vi "LSMcontroller_v57.vi"() -> ()   [LabVIEW 2015] (continued)
                    n4617 = local read "maxbufferAI"() -> (w1341:i32)
                    n4618 = local read "Override AI buffer"() -> (w1337:bool)
                    n4619 = call "2pparameters.vi"("command"="get") -> ("params out"=w1354:T12)  [unwired: 1 in]
                    n4620 = Bundle By Name(cluster=w1354, "type"="X-Y-t movie", "avpp"=w1357, "Angle Img"=w1356, "Xpixels Img"=w1352, "Vx-min Img"=w1351, "VX-max Img"=w1350, "Ypixels Img"=w1348, "Vy-min Img"=w1349, "Vy-max Img"=w1345, "srate"=w1339, "srate Img"=w1339, "finite"=w1340, "cont"=w1343, "wavdet"=w1344, "measpoints"=w1342, "maxbufferAI"=w1341, "Drawing Mode"=w1355, "Vz-reset"=0.0, "AIoverride"=w1337) -> (w1346:T12)
                    n4621 = call "2pparameters.vi"("Params in"=w1346, "command"="set") -> ()  [unwired: 1 out]
                  }
                  frame "X-Y-Z stack" {
                    n4622 = call "2pparameters.vi"("command"="get") -> ("params out"=w1361:T12)  [unwired: 1 in]
                    n4623 = Bundle By Name(cluster=w1361, "type"="X-Y-Z stack") -> (w1359:T12)
                    n4624 = call "2pparameters.vi"("Params in"=w1359, "command"="set") -> ()  [unwired: 1 out]
                  }
                  frame "Lifetime (scan)" {
                    n4625 = call "2pparameters.vi"("command"="get") -> ("params out"=w1366:T12)  [unwired: 1 in]
                    n4626 = Bundle By Name(cluster=w1366, "type"="Lifetime (scan)") -> (w1364:T12)
                    n4627 = call "2pparameters.vi"("Params in"=w1364, "command"="set") -> ()  [unwired: 1 out]
                  }
                  frame "Lifetime (contour)" {
                    n4628 = local read "Vy-min draw"() -> (w1376:dbl)
                    n4629 = local read "Vy-max draw"() -> (w1375:dbl)
                    n4630 = local read "Vx-min draw"() -> (w1378:dbl)
                    n4631 = local read "Vx-max draw"() -> (w1377:dbl)
                    n4632 = local read "xpixels ref"() -> (w1374:i32)
                    n4633 = local read "ypixels ref"() -> (w1373:i32)
                    n4634 = local read "ROI Type"() -> (w1372:u16)
                    n4635 = local read "srateAODOtt"() -> (w1383:dbl)
                    n4636 = local read "# of frames"() -> (w1388:i32)
                    n4637 = local read "refreshtime"() -> (w1380:dbl)
                    n4638 = local read "Pel"() -> (w1371:dbl)
                    n4639 = local read "bin"() -> (w1386:dbl)
                    n4640 = local read "Override AI buffer"() -> (w1369:bool)
                    n4641 = local read "finite samples"() -> (w1395:bool)
                    n4642 = local read "srateAODOtt"() -> (w1382:dbl)
                    n4643 = local read "srateAODOtt"() -> (w1389:dbl)
                    n4644 = local read "continuous"() -> (w1394:bool)
                    n4645 = local read "Angle ref"() -> (w1379:dbl)
                    n4646 = local read "wavdet"() -> (w1396:bool)
                    n4647 = local read "Vx-ref"() -> (w1391:dbl)
                    n4648 = local read "Vy-ref"() -> (w1393:dbl)
                    n4649 = local read "avpp"() -> (w1392:i32)
                    n4650 = call "tt_timeandsamples.vi"("bin"=w1386, "refreshtime"=w1380, "srateAODOtt"=w1383, "tot#ofsamples"=w1388) -> ("refreshrate"=w1384:dbl, "refreshbuffer"=w1385:i32, "timetracecycles"=w1390:i32)  [unwired: 5 in]
                    n4651 = local read "bin"() -> (w1387:dbl)
                    n4652 = call "2pparameters.vi"("command"="get") -> ("params out"=w1399:T12)  [unwired: 1 in]
                    n4653 = Bundle By Name(cluster=w1399, "Drawing Mode"=w1372, "measpoints"=w1388, "tt_cycles"=w1390, "refreshbuffer"=w1385, "refreshrate"=w1384, "Vx-ref"=w1391, "Vy-ref"=w1393, "srate"=w1382, "finite"=w1395, "cont"=w1394, "wavdet"=w1396, "avpp"=w1392, "srateAODO"=w1389, "bufferAI"=w1385, "bin"=w1387, "Angle Img"=w1379, "Vxminref"=w1378, "Vxmaxref"=w1377, "Vyminref"=w1376, "Vymaxref"=w1375, "Xpixels Img"=w1374, "Ypixels Img"=w1373, "Pel"=w1371, "Vz-reset"=0.0, "AIoverride"=w1369, "type"="Lifetime (contour)") -> (w1397:T12)
                    n4654 = Reciprocal(x=w1384) -> (1/x=w1381:dbl)
                    n4655 = local write "refreshtime"(w1381) -> ()
                    n4656 = call "2pparameters.vi"("Params in"=w1397, "command"="set") -> ()  [unwired: 1 out]
                  }
                  frame "X-Y-Z-t movie" {
                  }
                  frame "linescan" {
                  }
                  frame "Timetrace" {
                    n4657 = local read "Vy-min draw"() -> (w1409:dbl)
                    n4658 = local read "Vy-max draw"() -> (w1408:dbl)
                    n4659 = local read "Vx-min draw"() -> (w1411:dbl)
                    n4660 = local read "Vx-max draw"() -> (w1410:dbl)
                    n4661 = local read "xpixels ref"() -> (w1407:i32)
                    n4662 = local read "ypixels ref"() -> (w1406:i32)
                    n4663 = local read "ROI Type"() -> (w1405:u16)
                    n4664 = local read "srateAODOtt"() -> (w1416:dbl)
                    n4665 = local read "# of frames"() -> (w1421:i32)
                    n4666 = local read "refreshtime"() -> (w1413:dbl)
                    n4667 = local read "Pel"() -> (w1404:dbl)
                    n4668 = local read "bin"() -> (w1419:dbl)
                    n4669 = local read "Override AI buffer"() -> (w1402:bool)
                    n4670 = local read "finite samples"() -> (w1428:bool)
                    n4671 = local read "srateAODOtt"() -> (w1415:dbl)
                    n4672 = local read "srateAODOtt"() -> (w1422:dbl)
                    n4673 = local read "continuous"() -> (w1427:bool)
                    n4674 = local read "Angle ref"() -> (w1412:dbl)
                    n4675 = local read "wavdet"() -> (w1429:bool)
                    n4676 = local read "Vx-ref"() -> (w1424:dbl)
                    n4677 = local read "Vy-ref"() -> (w1426:dbl)
                    n4678 = local read "avpp"() -> (w1425:i32)
                    n4679 = call "tt_timeandsamples.vi"("bin"=w1419, "refreshtime"=w1413, "srateAODOtt"=w1416, "tot#ofsamples"=w1421) -> ("refreshrate"=w1417:dbl, "refreshbuffer"=w1418:i32, "timetracecycles"=w1423:i32)  [unwired: 5 in]
                    n4680 = local read "bin"() -> (w1420:dbl)
                    n4681 = call "2pparameters.vi"("command"="get") -> ("params out"=w1432:T12)  [unwired: 1 in]
                    n4682 = Bundle By Name(cluster=w1432, "Drawing Mode"=w1405, "measpoints"=w1421, "tt_cycles"=w1423, "refreshbuffer"=w1418, "refreshrate"=w1417, "Vx-ref"=w1424, "Vy-ref"=w1426, "srate"=w1415, "finite"=w1428, "cont"=w1427, "wavdet"=w1429, "avpp"=w1425, "srateAODO"=w1422, "bufferAI"=w1418, "bin"=w1420, "Angle Img"=w1412, "Vxminref"=w1411, "Vxmaxref"=w1410, "Vyminref"=w1409, "Vymaxref"=w1408, "Xpixels Img"=w1407, "Ypixels Img"=w1406, "Pel"=w1404, "Vz-reset"=0.0, "AIoverride"=w1402, "type"="Timetrace") -> (w1430:T12)
                    n4683 = Reciprocal(x=w1417) -> (1/x=w1414:dbl)
                    n4684 = local write "refreshtime"(w1414) -> ()
                    n4685 = call "2pparameters.vi"("Params in"=w1430, "command"="set") -> ()  [unwired: 1 out]
                  }
                  frame "Lifetime (point)" {
                  }
                }
              }
              frame #1 {
                w1435 = FALSE ("wavdet")
                n4686 = call "2pparameters.vi"("command"="get") -> ("params out"=w1439:T12)  [unwired: 1 in]
                n4687 = Bundle By Name(cluster=w1439, "finite"=w1435, "cont"=w1435, "wavdet"=TRUE) -> (w1436:T12)
                n4688 = call "2pparameters.vi"("Params in"=w1436, "command"="set") -> ()  [unwired: 1 out]
              }
              frame #2 {
                n4689 = local read "AO channels"() -> (w1444:u32)
                n4690 = call "2pparameters.vi"("command"="get") -> ("params out"=w1446:T12)  [unwired: 1 in]
                n4691 = Unbundle By Name(w1446) -> ("aAO"=w1445:u32[])
                n4692 = Search 1D Array(1D array=w1445, element=w1444) -> (index of element=w1442:i32)  [unwired: 1 in]
                n4693 = Greater?(x=w1442, y=-1) -> (0:w1441:bool)
                n4694 = case shown="True" w1441 {
                  tunnel: w1442 -> [_ w1456]
                  frame False {
                  }
                  frame True {
                    n4695 = local read "Meastab"() -> (w1449:enum32{"X-Y Image", "Linescan", "Timetrace"})
                    n4696 = local read "Tri padding value"() -> (w1450:dbl)
                    n4697 = local read "Amplitude (V)"() -> (w1454:dbl)
                    n4698 = local read "Tri Phase (s)"() -> (w1451:dbl)
                    n4699 = local read "Tri Repeats"() -> (w1452:dbl)
                    n4700 = local read "Frequency"() -> (w1453:dbl)
                    n4701 = local read "Offset (V)"() -> (w1455:dbl)
                    n4702 = case shown="\"Timetrace\"" w1449 {
                      tunnel: [w1457 w1458] -> w1448
                      frame "X-Y Image", Default {
                        n4703 = local read "Sampling rate"() -> (w1457:dbl)
                      }
                      frame "Timetrace" {
                        n4704 = local read "srateAODOtt"() -> (w1458:dbl)
                      }
                    }
                    n4705 = call "replace AO tri wf param.vi"("padding value"=w1450, "index of AO wave"=w1456, "Tri phase"=w1451, "Sampling frequency (Hz)"=w1448, "Tri Repeats"=w1452, "Frequency"=w1453, "Amplitude (V)"=w1454, "Offset (V)"=w1455) -> ()
                  }
                }
              }
              frame #3 {
                n4706 = case shown="True" w1459 {
                  tunnel: w1460 -> [_ w1469]
                  frame False {
                  }
                  frame True {
                    n4707 = call "waveformparamsv2.vi"("command"="get") -> ("Params out"=w1482:T16)  [unwired: 4 in, 2 out]
                    n4708 = Unbundle By Name(w1482) -> ("AO parameters"=w1481:T17)
                    n4709 = local read "Meastab"() -> (w1464:enum32{"X-Y Image", "Linescan", "Timetrace"})
                    n4710 = case shown="\"Timetrace\"" w1464 {
                      tunnel: [w1484 w1485] -> w1463
                      frame "X-Y Image", Default {
                        n4711 = local read "Sampling rate"() -> (w1484:dbl)
                      }
                      frame "Timetrace" {
                        n4712 = local read "srateAODOtt"() -> (w1485:dbl)
                      }
                    }
                    n4713 = Index Array(array=w1481, index=w1469) -> (element=w1471:T18)
                    n4714 = call "waveformsAObuffer.vi"("command"="get") -> ("AO wf out"=w1470:waveform(dbl)[])  [unwired: 1 in]
                    n4715 = call "generateTriWave_fromAOparameters.vi"("AO params"=w1471) -> ("Waveform"=w1468:waveform(dbl))  [unwired: 1 out]
                    n4716 = property on="refwf" class="Ring (strict)"() -> ("RingText.Text"=w1472:string)  [unwired: 2 in, 2 out]
                    n4717 = Replace Array Subset(array=w1470, new element=w1468, index=w1469) -> (w1467:waveform(dbl)[])
                    n4718 = call "waveformsDObuffer.vi"("command"="get") -> ("DO wf out"=w1477:digitalwaveform[])  [unwired: 1 in]
                    n4719 = call "correctwaveformsizetemp.vi"("new sampling frequency (Hz)"=w1463, "start"=FALSE, "reference waveforms to"=w1472, "Analog waveforms in"=w1467, "stop"=FALSE, "Digital waveforms in"=w1477) -> ("analog wf out"=w1475:waveform(dbl)[], "Digital wf out"=w1473:digitalwaveform[], "measpoints"=w1465:i32)
                    n4720 = local read "wavdet"() -> (w1466:bool)
                    n4721 = local write "Analog Lines Plot"(w1475) -> ()
                    n4722 = call "GetNumCamFramesv2.vi"("Digital Waveform Graph"=w1473) -> ("Numeric"=w1474:i32)  [unwired: 10 in]
                    n4723 = local write "Digital Lines Plot"(w1473) -> ()
                    n4724 = call "waveformsAObuffer.vi"("AO wf in"=w1475, "command"="set") -> ()  [unwired: 1 out]
                    n4725 = call "waveformsDObuffer.vi"("DO wf in"=w1473, "command"="set") -> ()  [unwired: 1 out]
                    n4726 = local write "Total Camera Frames"(w1474) -> ()
                    n4727 = case shown="True" w1466 {
                      tunnel: w1465 -> [_ w1486]
                      frame False {
                      }
                      frame True {
                        n4728 = local write "# of frames"(w1486) -> ()
                      }
                    }
                  }
                }
              }
              frame #4 {
                n4729 = local read "finite samples"() -> (w1487:bool)
                n4730 = local read "continuous"() -> (w1488:bool)
                n4731 = local read "wavdet"() -> (w1489:bool)
                n4732 = call "2pparameters.vi"("command"="get") -> ("params out"=w1492:T12)  [unwired: 1 in]
                n4733 = Bundle By Name(cluster=w1492, "finite"=w1487, "cont"=w1488, "wavdet"=w1489) -> (w1490:T12)
                n4734 = call "2pparameters.vi"("Params in"=w1490, "command"="set") -> ()  [unwired: 1 out]
              }
            }
          }
          event "Load Matlab Waveform": Value Change {
            n4735 = event-data() -> ()  [unwired: 1 in, 6 out]
            n4736 = stacked-sequence {
              seq-local: [_ _ w1600 _ _] -> [_ _ _ w1615 _]
              seq-local: [_ _ w1599 _ _] -> [_ _ _ w1614 _]
              frame #0 {
                n4737 = local read "Measurement"() -> (w1494:T5)
                n4738 = case shown="\"X-Y-t movie\", Default" w1494 {
                  frame "X-Y-t movie", Default {
                    n4739 = local read "avpp"() -> (w1515:i32)
                    n4740 = local read "Angle ref"() -> (w1514:dbl)
                    n4741 = local read "ROI Type"() -> (w1513:u16)
                    n4742 = local read "xpixels ref"() -> (w1510:i32)
                    n4743 = local read "Vx-min ref"() -> (w1509:dbl)
                    n4744 = local read "Vx-max ref"() -> (w1508:dbl)
                    n4745 = local read "ypixels ref"() -> (w1506:i32)
                    n4746 = local read "Vy-min ref"() -> (w1507:dbl)
                    n4747 = local read "Vy-max ref"() -> (w1503:dbl)
                    n4748 = local read "Sampling rate"() -> (w1497:dbl)
                    n4749 = local read "finite samples"() -> (w1498:bool)
                    n4750 = local read "continuous"() -> (w1501:bool)
                    n4751 = local read "wavdet"() -> (w1502:bool)
                    n4752 = local read "# of frames"() -> (w1500:i32)
                    n4753 = local read "maxbufferAI"() -> (w1499:i32)
                    n4754 = local read "Override AI buffer"() -> (w1495:bool)
                    n4755 = call "2pparameters.vi"("command"="get") -> ("params out"=w1512:T12)  [unwired: 1 in]
                    n4756 = Bundle By Name(cluster=w1512, "type"="X-Y-t movie", "avpp"=w1515, "Angle Img"=w1514, "Xpixels Img"=w1510, "Vx-min Img"=w1509, "VX-max Img"=w1508, "Ypixels Img"=w1506, "Vy-min Img"=w1507, "Vy-max Img"=w1503, "srate"=w1497, "srate Img"=w1497, "finite"=w1498, "cont"=w1501, "wavdet"=w1502, "measpoints"=w1500, "maxbufferAI"=w1499, "Drawing Mode"=w1513, "Vz-reset"=0.0, "AIoverride"=w1495) -> (w1504:T12)
                    n4757 = call "2pparameters.vi"("Params in"=w1504, "command"="set") -> ()  [unwired: 1 out]
                  }
                  frame "X-Y-Z stack" {
                    n4758 = call "2pparameters.vi"("command"="get") -> ("params out"=w1519:T12)  [unwired: 1 in]
                    n4759 = Bundle By Name(cluster=w1519, "type"="X-Y-Z stack") -> (w1517:T12)
                    n4760 = call "2pparameters.vi"("Params in"=w1517, "command"="set") -> ()  [unwired: 1 out]
                  }
                  frame "Lifetime (scan)" {
                    n4761 = call "2pparameters.vi"("command"="get") -> ("params out"=w1524:T12)  [unwired: 1 in]
                    n4762 = Bundle By Name(cluster=w1524, "type"="Lifetime (scan)") -> (w1522:T12)
                    n4763 = call "2pparameters.vi"("Params in"=w1522, "command"="set") -> ()  [unwired: 1 out]
                  }
                  frame "Lifetime (contour)" {
                    n4764 = local read "Vy-min draw"() -> (w1534:dbl)
                    n4765 = local read "Vy-max draw"() -> (w1533:dbl)
                    n4766 = local read "Vx-min draw"() -> (w1536:dbl)
                    n4767 = local read "Vx-max draw"() -> (w1535:dbl)
                    n4768 = local read "xpixels ref"() -> (w1532:i32)
                    n4769 = local read "ypixels ref"() -> (w1531:i32)
                    n4770 = local read "ROI Type"() -> (w1530:u16)
                    n4771 = local read "srateAODOtt"() -> (w1541:dbl)
                    n4772 = local read "# of frames"() -> (w1546:i32)
                    n4773 = local read "refreshtime"() -> (w1538:dbl)
                    n4774 = local read "Pel"() -> (w1529:dbl)
                    n4775 = local read "bin"() -> (w1544:dbl)
                    n4776 = local read "Override AI buffer"() -> (w1527:bool)
                    n4777 = local read "finite samples"() -> (w1553:bool)
                    n4778 = local read "srateAODOtt"() -> (w1540:dbl)
                    n4779 = local read "srateAODOtt"() -> (w1547:dbl)
                    n4780 = local read "continuous"() -> (w1552:bool)
                    n4781 = local read "Angle ref"() -> (w1537:dbl)
                    n4782 = local read "wavdet"() -> (w1554:bool)
                    n4783 = local read "Vx-ref"() -> (w1549:dbl)
                    n4784 = local read "Vy-ref"() -> (w1551:dbl)
                    n4785 = local read "avpp"() -> (w1550:i32)
                    n4786 = call "tt_timeandsamples.vi"("bin"=w1544, "refreshtime"=w1538, "srateAODOtt"=w1541, "tot#ofsamples"=w1546) -> ("refreshrate"=w1542:dbl, "refreshbuffer"=w1543:i32, "timetracecycles"=w1548:i32)  [unwired: 5 in]
                    n4787 = local read "bin"() -> (w1545:dbl)
                    n4788 = call "2pparameters.vi"("command"="get") -> ("params out"=w1557:T12)  [unwired: 1 in]
                    n4789 = Bundle By Name(cluster=w1557, "Drawing Mode"=w1530, "measpoints"=w1546, "tt_cycles"=w1548, "refreshbuffer"=w1543, "refreshrate"=w1542, "Vx-ref"=w1549, "Vy-ref"=w1551, "srate"=w1540, "finite"=w1553, "cont"=w1552, "wavdet"=w1554, "avpp"=w1550, "srateAODO"=w1547, "bufferAI"=w1543, "bin"=w1545, "Angle Img"=w1537, "Vxminref"=w1536, "Vxmaxref"=w1535, "Vyminref"=w1534, "Vymaxref"=w1533, "Xpixels Img"=w1532, "Ypixels Img"=w1531, "Pel"=w1529, "Vz-reset"=0.0, "AIoverride"=w1527, "type"="Lifetime (contour)") -> (w1555:T12)
                    n4790 = Reciprocal(x=w1542) -> (1/x=w1539:dbl)
                    n4791 = local write "refreshtime"(w1539) -> ()
                    n4792 = call "2pparameters.vi"("Params in"=w1555, "command"="set") -> ()  [unwired: 1 out]
                  }
                  frame "X-Y-Z-t movie" {
                  }
                  frame "linescan" {
                  }
                  frame "Timetrace" {
                    n4793 = local read "Vy-min draw"() -> (w1567:dbl)
                    n4794 = local read "Vy-max draw"() -> (w1566:dbl)
                    n4795 = local read "Vx-min draw"() -> (w1569:dbl)
                    n4796 = local read "Vx-max draw"() -> (w1568:dbl)
                    n4797 = local read "xpixels ref"() -> (w1565:i32)
                    n4798 = local read "ypixels ref"() -> (w1564:i32)
                    n4799 = local read "ROI Type"() -> (w1563:u16)
                    n4800 = local read "srateAODOtt"() -> (w1574:dbl)
                    n4801 = local read "# of frames"() -> (w1579:i32)
                    n4802 = local read "refreshtime"() -> (w1571:dbl)
                    n4803 = local read "Pel"() -> (w1562:dbl)
                    n4804 = local read "bin"() -> (w1577:dbl)
                    n4805 = local read "Override AI buffer"() -> (w1560:bool)
                    n4806 = local read "finite samples"() -> (w1586:bool)
                    n4807 = local read "srateAODOtt"() -> (w1573:dbl)
                    n4808 = local read "srateAODOtt"() -> (w1580:dbl)
                    n4809 = local read "continuous"() -> (w1585:bool)
                    n4810 = local read "Angle ref"() -> (w1570:dbl)
                    n4811 = local read "wavdet"() -> (w1587:bool)
                    n4812 = local read "Vx-ref"() -> (w1582:dbl)
                    n4813 = local read "Vy-ref"() -> (w1584:dbl)
                    n4814 = local read "avpp"() -> (w1583:i32)
                    n4815 = call "tt_timeandsamples.vi"("bin"=w1577, "refreshtime"=w1571, "srateAODOtt"=w1574, "tot#ofsamples"=w1579) -> ("refreshrate"=w1575:dbl, "refreshbuffer"=w1576:i32, "timetracecycles"=w1581:i32)  [unwired: 5 in]
                    n4816 = local read "bin"() -> (w1578:dbl)
                    n4817 = call "2pparameters.vi"("command"="get") -> ("params out"=w1590:T12)  [unwired: 1 in]
                    n4818 = Bundle By Name(cluster=w1590, "Drawing Mode"=w1563, "measpoints"=w1579, "tt_cycles"=w1581, "refreshbuffer"=w1576, "refreshrate"=w1575, "Vx-ref"=w1582, "Vy-ref"=w1584, "srate"=w1573, "finite"=w1586, "cont"=w1585, "wavdet"=w1587, "avpp"=w1583, "srateAODO"=w1580, "bufferAI"=w1576, "bin"=w1578, "Angle Img"=w1570, "Vxminref"=w1569, "Vxmaxref"=w1568, "Vyminref"=w1567, "Vymaxref"=w1566, "Xpixels Img"=w1565, "Ypixels Img"=w1564, "Pel"=w1562, "Vz-reset"=0.0, "AIoverride"=w1560, "type"="Timetrace") -> (w1588:T12)
                    n4819 = Reciprocal(x=w1575) -> (1/x=w1572:dbl)
                    n4820 = local write "refreshtime"(w1572) -> ()
                    n4821 = call "2pparameters.vi"("Params in"=w1588, "command"="set") -> ()  [unwired: 1 out]
                  }
                  frame "Lifetime (point)" {
                  }
                }
              }
              frame #1 {
                w1593 = FALSE ("wavdet")
                n4822 = call "2pparameters.vi"("command"="get") -> ("params out"=w1597:T12)  [unwired: 1 in]
                n4823 = Bundle By Name(cluster=w1597, "finite"=w1593, "cont"=w1593, "wavdet"=TRUE) -> (w1594:T12)
                n4824 = call "2pparameters.vi"("Params in"=w1594, "command"="set") -> ()  [unwired: 1 out]
              }
              frame #2 {
                n4825 = local read "AO channels"() -> (w1602:u32)
                n4826 = call "2pparameters.vi"("command"="get") -> ("params out"=w1604:T12)  [unwired: 1 in]
                n4827 = Unbundle By Name(w1604) -> ("aAO"=w1603:u32[])
                n4828 = Search 1D Array(1D array=w1603, element=w1602) -> (index of element=w1600:i32)  [unwired: 1 in]
                n4829 = Greater?(x=w1600, y=-1) -> (0:w1599:bool)
                n4830 = case shown="True" w1599 {
                  tunnel: w1600 -> [_ w1611]
                  frame False {
                  }
                  frame True {
                    n4831 = local read "Meastab"() -> (w1607:enum32{"X-Y Image", "Linescan", "Timetrace"})
                    n4832 = local read "Matlab waveform path"() -> (w1609:path)
                    n4833 = local read "Matlab padding value"() -> (w1610:dbl)
                    n4834 = case shown="\"Timetrace\"" w1607 {
                      tunnel: [w1612 w1613] -> w1606
                      frame "X-Y Image", Default {
                        n4835 = local read "Sampling rate"() -> (w1612:dbl)
                      }
                      frame "Timetrace" {
                        n4836 = local read "srateAODOtt"() -> (w1613:dbl)
                      }
                    }
                    n4837 = call "matlabwfexistsdialogue.vi"("Matlab waveform path"=w1609) -> ("mtalab waveform path out"=w1608:path)
                    n4838 = call "replace AO matlab param.vi"("Sampling frequency (Hz)"=w1606, "matlab wave file"=w1608, "index of AO wave"=w1611, "padding value"=w1610) -> ()  [unwired: 7 in]
                  }
                }
              }
              frame #3 {
                n4839 = case shown="True" w1614 {
                  tunnel: w1615 -> [_ w1622]
                  frame False {
                  }
                  frame True {
                    n4840 = local read "Meastab"() -> (w1619:enum32{"X-Y Image", "Linescan", "Timetrace"})
                    n4841 = call "waveformparamsv2.vi"("command"="get") -> ("Params out"=w1625:T16)  [unwired: 4 in, 2 out]
                    n4842 = Unbundle By Name(w1625) -> ("AO parameters"=w1624:T17)
                    n4843 = case shown="\"Timetrace\"" w1619 {
                      tunnel: [w1639 w1640] -> w1618
                      frame "X-Y Image", Default {
                        n4844 = local read "Sampling rate"() -> (w1639:dbl)
                      }
                      frame "Timetrace" {
                        n4845 = local read "srateAODOtt"() -> (w1640:dbl)
                      }
                    }
                    n4846 = Index Array(array=w1624, index=w1622) -> (element=w1623:T18)
                    n4847 = call "waveformsAObuffer.vi"("command"="get") -> ("AO wf out"=w1629:waveform(dbl)[])  [unwired: 1 in]
                    n4848 = call "matlabAOwffromparam.vi"("Cluster"=w1623) -> ("Waveform"=w1627:waveform(dbl))  [unwired: 1 out]
                    n4849 = property on="refwf" class="Ring (strict)"() -> ("RingText.Text"=w1630:string)  [unwired: 2 in, 2 out]
                    n4850 = Replace Array Subset(array=w1629, new element=w1627, index=w1622) -> (w1628:waveform(dbl)[])
                    n4851 = call "waveformsDObuffer.vi"("command"="get") -> ("DO wf out"=w1635:digitalwaveform[])  [unwired: 1 in]
                    n4852 = call "correctwaveformsizetemp.vi"("new sampling frequency (Hz)"=w1618, "start"=FALSE, "reference waveforms to"=w1630, "Analog waveforms in"=w1628, "stop"=FALSE, "Digital waveforms in"=w1635) -> ("analog wf out"=w1633:waveform(dbl)[], "Digital wf out"=w1631:digitalwaveform[], "measpoints"=w1620:i32)
                    n4853 = local read "wavdet"() -> (w1621:bool)
                    n4854 = local write "Analog Lines Plot"(w1633) -> ()
                    n4855 = call "GetNumCamFramesv2.vi"("Digital Waveform Graph"=w1631) -> ("Numeric"=w1632:i32)  [unwired: 10 in]
                    n4856 = local write "Digital Lines Plot"(w1631) -> ()
                    n4857 = call "waveformsAObuffer.vi"("AO wf in"=w1633, "command"="set") -> ()  [unwired: 1 out]
                    n4858 = call "waveformsDObuffer.vi"("DO wf in"=w1631, "command"="set") -> ()  [unwired: 1 out]
                    n4859 = local write "Total Camera Frames"(w1632) -> ()
                    n4860 = case shown="True" w1621 {
                      tunnel: w1620 -> [_ w1641]
                      frame False {
                      }
                      frame True {
                        n4861 = local write "# of frames"(w1641) -> ()
                      }
                    }
                  }
                }
              }
              frame #4 {
                n4862 = local read "finite samples"() -> (w1642:bool)
                n4863 = local read "continuous"() -> (w1643:bool)
                n4864 = local read "wavdet"() -> (w1644:bool)
                n4865 = call "2pparameters.vi"("command"="get") -> ("params out"=w1647:T12)  [unwired: 1 in]
                n4866 = Bundle By Name(cluster=w1647, "finite"=w1642, "cont"=w1643, "wavdet"=w1644) -> (w1645:T12)
                n4867 = call "2pparameters.vi"("Params in"=w1645, "command"="set") -> ()  [unwired: 1 out]
              }
            }
          }
          event "Load Matlab Waveform DO": Value Change {
            n4868 = event-data() -> ()  [unwired: 1 in, 6 out]
            n4869 = stacked-sequence {
              seq-local: [_ _ w1755 _ _] -> [_ _ _ w1770 _]
              seq-local: [_ _ w1754 _ _] -> [_ _ _ w1769 _]
              frame #0 {
                n4870 = local read "Measurement"() -> (w1649:T5)
                n4871 = case shown="\"X-Y-t movie\", Default" w1649 {
                  frame "X-Y-t movie", Default {
                    n4872 = local read "avpp"() -> (w1670:i32)
                    n4873 = local read "Angle ref"() -> (w1669:dbl)
                    n4874 = local read "ROI Type"() -> (w1668:u16)
                    n4875 = local read "xpixels ref"() -> (w1665:i32)
                    n4876 = local read "Vx-min ref"() -> (w1664:dbl)
                    n4877 = local read "Vx-max ref"() -> (w1663:dbl)
                    n4878 = local read "ypixels ref"() -> (w1661:i32)
                    n4879 = local read "Vy-min ref"() -> (w1662:dbl)
                    n4880 = local read "Vy-max ref"() -> (w1658:dbl)
                    n4881 = local read "Sampling rate"() -> (w1652:dbl)
                    n4882 = local read "finite samples"() -> (w1653:bool)
                    n4883 = local read "continuous"() -> (w1656:bool)
                    n4884 = local read "wavdet"() -> (w1657:bool)
                    n4885 = local read "# of frames"() -> (w1655:i32)
                    n4886 = local read "maxbufferAI"() -> (w1654:i32)
                    n4887 = local read "Override AI buffer"() -> (w1650:bool)
                    n4888 = call "2pparameters.vi"("command"="get") -> ("params out"=w1667:T12)  [unwired: 1 in]
                    n4889 = Bundle By Name(cluster=w1667, "type"="X-Y-t movie", "avpp"=w1670, "Angle Img"=w1669, "Xpixels Img"=w1665, "Vx-min Img"=w1664, "VX-max Img"=w1663, "Ypixels Img"=w1661, "Vy-min Img"=w1662, "Vy-max Img"=w1658, "srate"=w1652, "srate Img"=w1652, "finite"=w1653, "cont"=w1656, "wavdet"=w1657, "measpoints"=w1655, "maxbufferAI"=w1654, "Drawing Mode"=w1668, "Vz-reset"=0.0, "AIoverride"=w1650) -> (w1659:T12)
                    n4890 = call "2pparameters.vi"("Params in"=w1659, "command"="set") -> ()  [unwired: 1 out]
                  }
                  frame "X-Y-Z stack" {
                    n4891 = call "2pparameters.vi"("command"="get") -> ("params out"=w1674:T12)  [unwired: 1 in]
                    n4892 = Bundle By Name(cluster=w1674, "type"="X-Y-Z stack") -> (w1672:T12)
                    n4893 = call "2pparameters.vi"("Params in"=w1672, "command"="set") -> ()  [unwired: 1 out]
                  }
                  frame "Lifetime (scan)" {
                    n4894 = call "2pparameters.vi"("command"="get") -> ("params out"=w1679:T12)  [unwired: 1 in]
                    n4895 = Bundle By Name(cluster=w1679, "type"="Lifetime (scan)") -> (w1677:T12)
                    n4896 = call "2pparameters.vi"("Params in"=w1677, "command"="set") -> ()  [unwired: 1 out]
                  }
                  frame "Lifetime (contour)" {
                    n4897 = local read "Vy-min draw"() -> (w1689:dbl)
                    n4898 = local read "Vy-max draw"() -> (w1688:dbl)
                    n4899 = local read "Vx-min draw"() -> (w1691:dbl)
                    n4900 = local read "Vx-max draw"() -> (w1690:dbl)
                    n4901 = local read "xpixels ref"() -> (w1687:i32)
                    n4902 = local read "ypixels ref"() -> (w1686:i32)
                    n4903 = local read "ROI Type"() -> (w1685:u16)
                    n4904 = local read "srateAODOtt"() -> (w1696:dbl)
                    n4905 = local read "# of frames"() -> (w1701:i32)
                    n4906 = local read "refreshtime"() -> (w1693:dbl)
                    n4907 = local read "Pel"() -> (w1684:dbl)
                    n4908 = local read "bin"() -> (w1699:dbl)
                    n4909 = local read "Override AI buffer"() -> (w1682:bool)
                    n4910 = local read "finite samples"() -> (w1708:bool)
                    n4911 = local read "srateAODOtt"() -> (w1695:dbl)
                    n4912 = local read "srateAODOtt"() -> (w1702:dbl)
                    n4913 = local read "continuous"() -> (w1707:bool)
                    n4914 = local read "Angle ref"() -> (w1692:dbl)
                    n4915 = local read "wavdet"() -> (w1709:bool)
                    n4916 = local read "Vx-ref"() -> (w1704:dbl)
                    n4917 = local read "Vy-ref"() -> (w1706:dbl)
                    n4918 = local read "avpp"() -> (w1705:i32)
                    n4919 = call "tt_timeandsamples.vi"("bin"=w1699, "refreshtime"=w1693, "srateAODOtt"=w1696, "tot#ofsamples"=w1701) -> ("refreshrate"=w1697:dbl, "refreshbuffer"=w1698:i32, "timetracecycles"=w1703:i32)  [unwired: 5 in]
                    n4920 = local read "bin"() -> (w1700:dbl)
                    n4921 = call "2pparameters.vi"("command"="get") -> ("params out"=w1712:T12)  [unwired: 1 in]
                    n4922 = Bundle By Name(cluster=w1712, "Drawing Mode"=w1685, "measpoints"=w1701, "tt_cycles"=w1703, "refreshbuffer"=w1698, "refreshrate"=w1697, "Vx-ref"=w1704, "Vy-ref"=w1706, "srate"=w1695, "finite"=w1708, "cont"=w1707, "wavdet"=w1709, "avpp"=w1705, "srateAODO"=w1702, "bufferAI"=w1698, "bin"=w1700, "Angle Img"=w1692, "Vxminref"=w1691, "Vxmaxref"=w1690, "Vyminref"=w1689, "Vymaxref"=w1688, "Xpixels Img"=w1687, "Ypixels Img"=w1686, "Pel"=w1684, "Vz-reset"=0.0, "AIoverride"=w1682, "type"="Lifetime (contour)") -> (w1710:T12)
                    n4923 = Reciprocal(x=w1697) -> (1/x=w1694:dbl)
                    n4924 = local write "refreshtime"(w1694) -> ()
                    n4925 = call "2pparameters.vi"("Params in"=w1710, "command"="set") -> ()  [unwired: 1 out]
                  }
                  frame "X-Y-Z-t movie" {
                  }
                  frame "linescan" {
                  }
                  frame "Timetrace" {
                    n4926 = local read "Vy-min draw"() -> (w1722:dbl)
                    n4927 = local read "Vy-max draw"() -> (w1721:dbl)
                    n4928 = local read "Vx-min draw"() -> (w1724:dbl)
                    n4929 = local read "Vx-max draw"() -> (w1723:dbl)
                    n4930 = local read "xpixels ref"() -> (w1720:i32)
                    n4931 = local read "ypixels ref"() -> (w1719:i32)
                    n4932 = local read "ROI Type"() -> (w1718:u16)
                    n4933 = local read "srateAODOtt"() -> (w1729:dbl)
                    n4934 = local read "# of frames"() -> (w1734:i32)
                    n4935 = local read "refreshtime"() -> (w1726:dbl)
                    n4936 = local read "Pel"() -> (w1717:dbl)
                    n4937 = local read "bin"() -> (w1732:dbl)
                    n4938 = local read "Override AI buffer"() -> (w1715:bool)
                    n4939 = local read "finite samples"() -> (w1741:bool)
                    n4940 = local read "srateAODOtt"() -> (w1728:dbl)
                    n4941 = local read "srateAODOtt"() -> (w1735:dbl)
                    n4942 = local read "continuous"() -> (w1740:bool)
                    n4943 = local read "Angle ref"() -> (w1725:dbl)
                    n4944 = local read "wavdet"() -> (w1742:bool)
                    n4945 = local read "Vx-ref"() -> (w1737:dbl)
                    n4946 = local read "Vy-ref"() -> (w1739:dbl)
                    n4947 = local read "avpp"() -> (w1738:i32)
                    n4948 = call "tt_timeandsamples.vi"("bin"=w1732, "refreshtime"=w1726, "srateAODOtt"=w1729, "tot#ofsamples"=w1734) -> ("refreshrate"=w1730:dbl, "refreshbuffer"=w1731:i32, "timetracecycles"=w1736:i32)  [unwired: 5 in]
                    n4949 = local read "bin"() -> (w1733:dbl)
                    n4950 = call "2pparameters.vi"("command"="get") -> ("params out"=w1745:T12)  [unwired: 1 in]
                    n4951 = Bundle By Name(cluster=w1745, "Drawing Mode"=w1718, "measpoints"=w1734, "tt_cycles"=w1736, "refreshbuffer"=w1731, "refreshrate"=w1730, "Vx-ref"=w1737, "Vy-ref"=w1739, "srate"=w1728, "finite"=w1741, "cont"=w1740, "wavdet"=w1742, "avpp"=w1738, "srateAODO"=w1735, "bufferAI"=w1731, "bin"=w1733, "Angle Img"=w1725, "Vxminref"=w1724, "Vxmaxref"=w1723, "Vyminref"=w1722, "Vymaxref"=w1721, "Xpixels Img"=w1720, "Ypixels Img"=w1719, "Pel"=w1717, "Vz-reset"=0.0, "AIoverride"=w1715, "type"="Timetrace") -> (w1743:T12)
                    n4952 = Reciprocal(x=w1730) -> (1/x=w1727:dbl)
                    n4953 = local write "refreshtime"(w1727) -> ()
                    n4954 = call "2pparameters.vi"("Params in"=w1743, "command"="set") -> ()  [unwired: 1 out]
                  }
                  frame "Lifetime (point)" {
                  }
                }
              }
              frame #1 {
                w1748 = FALSE ("wavdet")
                n4955 = call "2pparameters.vi"("command"="get") -> ("params out"=w1752:T12)  [unwired: 1 in]
                n4956 = Bundle By Name(cluster=w1752, "finite"=w1748, "cont"=w1748, "wavdet"=TRUE) -> (w1749:T12)
                n4957 = call "2pparameters.vi"("Params in"=w1749, "command"="set") -> ()  [unwired: 1 out]
              }
              frame #2 {
                n4958 = local read "DO channels"() -> (w1757:u16)
                n4959 = call "2pparameters.vi"("command"="get") -> ("params out"=w1759:T12)  [unwired: 1 in]
                n4960 = Unbundle By Name(w1759) -> ("aDO"=w1758:u32[])
                n4961 = Search 1D Array(1D array=w1758, element=w1757) -> (index of element=w1755:i32)  [unwired: 1 in]
                n4962 = Greater?(x=w1755, y=-1) -> (0:w1754:bool)
                n4963 = case shown="True" w1754 {
                  tunnel: w1755 -> [_ w1766]
                  frame False {
                  }
                  frame True {
                    n4964 = local read "Meastab"() -> (w1762:enum32{"X-Y Image", "Linescan", "Timetrace"})
                    n4965 = local read "Matlab waveform path DO"() -> (w1764:path)
                    n4966 = local read "Matlab padding value DO"() -> (w1765:dbl)
                    n4967 = case shown="\"Timetrace\"" w1762 {
                      tunnel: [w1767 w1768] -> w1761
                      frame "X-Y Image", Default {
                        n4968 = local read "Sampling rate"() -> (w1767:dbl)
                      }
                      frame "Timetrace" {
                        n4969 = local read "srateAODOtt"() -> (w1768:dbl)
                      }
                    }
                    n4970 = call "matlabwfexistsdialogue.vi"("Matlab waveform path"=w1764) -> ("mtalab waveform path out"=w1763:path)
                    n4971 = call "replace DO matlab param.vi"("Sampling frequency (Hz)"=w1761, "matlab wave number"=w1763, "index of DO wave"=w1766, "padding value"=w1765) -> ()  [unwired: 7 in]
                  }
                }
              }
              frame #3 {
                n4972 = case shown="True" w1769 {
                  tunnel: w1770 -> [_ w1779]
                  frame False {
                  }
                  frame True {
                    n4973 = local read "Meastab"() -> (w1774:enum32{"X-Y Image", "Linescan", "Timetrace"})
                    n4974 = call "waveformparamsv2.vi"("command"="get") -> ("Params out"=w1792:T16)  [unwired: 4 in, 2 out]
                    n4975 = Unbundle By Name(w1792) -> ("DO parameters"=w1791:T19)
                    n4976 = case shown="\"Timetrace\"" w1774 {
                      tunnel: [w1794 w1795] -> w1773
                      frame "X-Y Image", Default {
                        n4977 = local read "Sampling rate"() -> (w1794:dbl)
                      }
                      frame "Timetrace" {
                        n4978 = local read "srateAODOtt"() -> (w1795:dbl)
                      }
                    }
                    n4979 = Index Array(array=w1791, index=w1779) -> (element=w1778:T20)
                    n4980 = call "waveformsDObuffer.vi"("command"="get") -> ("DO wf out"=w1789:digitalwaveform[])  [unwired: 1 in]
                    n4981 = property on="refwf" class="Ring (strict)"() -> ("RingText.Text"=w1781:string)  [unwired: 2 in, 2 out]
                    n4982 = call "matlabDOwffromparam.vi"("waveform params"=w1778) -> ("digital waveform"=w1777:digitalwaveform)
                    n4983 = Replace Array Subset(array=w1789, new element=w1777, index=w1779) -> (w1780:digitalwaveform[])
                    n4984 = call "waveformsAObuffer.vi"("command"="get") -> ("AO wf out"=w1788:waveform(dbl)[])  [unwired: 1 in]
                    n4985 = local read "wavdet"() -> (w1776:bool)
                    n4986 = call "correctwaveformsizetemp.vi"("new sampling frequency (Hz)"=w1773, "start"=FALSE, "reference waveforms to"=w1781, "Analog waveforms in"=w1788, "stop"=FALSE, "Digital waveforms in"=w1780) -> ("analog wf out"=w1784:waveform(dbl)[], "Digital wf out"=w1782:digitalwaveform[], "measpoints"=w1775:i32)
                    n4987 = local write "Analog Lines Plot"(w1784) -> ()
                    n4988 = call "GetNumCamFramesv2.vi"("Digital Waveform Graph"=w1782) -> ("Numeric"=w1783:i32)  [unwired: 10 in]
                    n4989 = local write "Digital Lines Plot"(w1782) -> ()
                    n4990 = case shown="True" w1776 {
                      tunnel: w1775 -> [_ w1796]
                      frame False {
                      }
                      frame True {
                        n4991 = local write "# of frames"(w1796) -> ()
                      }
                    }
                    n4992 = call "waveformsAObuffer.vi"("AO wf in"=w1784, "command"="set") -> ()  [unwired: 1 out]
                    n4993 = call "waveformsDObuffer.vi"("DO wf in"=w1782, "command"="set") -> ()  [unwired: 1 out]
                    n4994 = local write "Total Camera Frames"(w1783) -> ()
                  }
                }
              }
              frame #4 {
                n4995 = local read "finite samples"() -> (w1797:bool)
                n4996 = local read "continuous"() -> (w1798:bool)
                n4997 = local read "wavdet"() -> (w1799:bool)
                n4998 = call "2pparameters.vi"("command"="get") -> ("params out"=w1802:T12)  [unwired: 1 in]
                n4999 = Bundle By Name(cluster=w1802, "finite"=w1797, "cont"=w1798, "wavdet"=w1799) -> (w1800:T12)
                n5000 = call "2pparameters.vi"("Params in"=w1800, "command"="set") -> ()  [unwired: 1 out]
              }
            }
          }
          event "Add settings": Value Change {
            n5001 = event-data() -> ()  [unwired: 1 in, 6 out]
            n5002 = call "wfsettings.vi"("command"="get") -> ("wfsettings out"=w1806:T29)  [unwired: 2 in, 1 out]
            n5003 = in-place {
              n5004 = in-place-cluster #53(w1806) -> ("settings names"=w1811:string[], "settings locations"=w1813:path[])
              n5005 = local read "Setting location"() -> (w1809:path)
              n5006 = local read "Nickname"() -> (w1808:string)
              n5007 = Build Array (concatenate)(w1811, w1808) -> (w1810:string[])
              n5008 = property on="Loaded settings" class="Ring (strict)"("Strings []"=w1810) -> ()  [unwired: 2 in, 2 out]
              n5009 = Build Array (concatenate)(w1813, w1809) -> (w1812:path[])
              n5010 = in-place-cluster #53("settings names"=w1810, "settings locations"=w1812) -> (w1804:T29)
            }
            n5011 = call "wfsettings.vi"("wfsettings in"=w1804, "command"="set") -> ()  [unwired: 1 in, 2 out]
          }
          event "Rem setting": Value Change {
            n5012 = event-data() -> ()  [unwired: 1 in, 6 out]
            n5013 = call "wfsettings.vi"("command"="get") -> ("wfsettings out"=w1816:T29)  [unwired: 2 in, 1 out]
            n5014 = in-place {
              n5015 = in-place-cluster #54(w1816) -> ("settings names"=w1821:string[], "settings locations"=w1819:path[])
              n5016 = property on="Loaded settings" class="Ring (strict)"() -> ("RingText.Text"=w1822:string)  [unwired: 2 in, 2 out]
              n5017 = Search 1D Array(1D array=w1821, element=w1822) -> (index of element=w1823:i32)  [unwired: 1 in]
              n5018 = Delete From Array(array=w1821, index=w1823) -> (array with subset deleted=w1820:string[])  [unwired: 1 in, 1 out]
              n5019 = Delete From Array(array=w1819, index=w1823) -> (array with subset deleted=w1818:path[])  [unwired: 1 in, 1 out]
              n5020 = property on="Loaded settings" class="Ring (strict)"("Strings []"=w1820) -> ()  [unwired: 2 in, 2 out]
              n5021 = in-place-cluster #54("settings names"=w1820, "settings locations"=w1818) -> (w1814:T29)
            }
            n5022 = call "wfsettings.vi"("wfsettings in"=w1814, "command"="set") -> ()  [unwired: 1 in, 2 out]
          }
          event "Update settings": Value Change {
            n5023 = event-data() -> ()  [unwired: 1 in, 6 out]
            n5024 = stacked-sequence {
              frame #0 {
                n5025 = local read "Measurement"() -> (w1824:T5)
                n5026 = case shown="\"Timetrace\"" w1824 {
                  frame "X-Y-t movie", Default {
                    n5027 = local read "avpp"() -> (w1845:i32)
                    n5028 = local read "Angle ref"() -> (w1844:dbl)
                    n5029 = local read "ROI Type"() -> (w1843:u16)
                    n5030 = local read "xpixels ref"() -> (w1840:i32)
                    n5031 = local read "Vx-min ref"() -> (w1839:dbl)
                    n5032 = local read "Vx-max ref"() -> (w1838:dbl)
                    n5033 = local read "ypixels ref"() -> (w1836:i32)
                    n5034 = local read "Vy-min ref"() -> (w1837:dbl)
                    n5035 = local read "Vy-max ref"() -> (w1833:dbl)
                    n5036 = local read "Sampling rate"() -> (w1827:dbl)
                    n5037 = local read "finite samples"() -> (w1828:bool)
                    n5038 = local read "continuous"() -> (w1831:bool)
                    n5039 = local read "wavdet"() -> (w1832:bool)
                    n5040 = local read "# of frames"() -> (w1830:i32)
                    n5041 = local read "maxbufferAI"() -> (w1829:i32)
                    n5042 = local read "Override AI buffer"() -> (w1825:bool)
                    n5043 = call "2pparameters.vi"("command"="get") -> ("params out"=w1842:T12)  [unwired: 1 in]
                    n5044 = Bundle By Name(cluster=w1842, "type"="X-Y-t movie", "avpp"=w1845, "Angle Img"=w1844, "Xpixels Img"=w1840, "Vx-min Img"=w1839, "VX-max Img"=w1838, "Ypixels Img"=w1836, "Vy-min Img"=w1837, "Vy-max Img"=w1833, "srate"=w1827, "srate Img"=w1827, "finite"=w1828, "cont"=w1831, "wavdet"=w1832, "measpoints"=w1830, "maxbufferAI"=w1829, "Drawing Mode"=w1843, "Vz-reset"=0.0, "AIoverride"=w1825) -> (w1834:T12)
                    n5045 = call "2pparameters.vi"("Params in"=w1834, "command"="set") -> ()  [unwired: 1 out]
                  }
                  frame "X-Y-Z stack" {
                    n5046 = call "2pparameters.vi"("command"="get") -> ("params out"=w1849:T12)  [unwired: 1 in]
                    n5047 = Bundle By Name(cluster=w1849, "type"="X-Y-Z stack") -> (w1847:T12)
                    n5048 = call "2pparameters.vi"("Params in"=w1847, "command"="set") -> ()  [unwired: 1 out]
                  }
                  frame "Lifetime (scan)" {
                    n5049 = call "2pparameters.vi"("command"="get") -> ("params out"=w1854:T12)  [unwired: 1 in]
                    n5050 = Bundle By Name(cluster=w1854, "type"="Lifetime (scan)") -> (w1852:T12)
                    n5051 = call "2pparameters.vi"("Params in"=w1852, "command"="set") -> ()  [unwired: 1 out]
                  }
                  frame "Lifetime (contour)" {
                    n5052 = local read "Vy-min draw"() -> (w1864:dbl)
                    n5053 = local read "Vy-max draw"() -> (w1863:dbl)
                    n5054 = local read "Vx-min draw"() -> (w1866:dbl)
                    n5055 = local read "Vx-max draw"() -> (w1865:dbl)
                    n5056 = local read "xpixels ref"() -> (w1862:i32)
                    n5057 = local read "ypixels ref"() -> (w1861:i32)
                    n5058 = local read "ROI Type"() -> (w1860:u16)
                    n5059 = local read "srateAODOtt"() -> (w1871:dbl)
                    n5060 = local read "# of frames"() -> (w1876:i32)
                    n5061 = local read "refreshtime"() -> (w1868:dbl)
                    n5062 = local read "Pel"() -> (w1859:dbl)
                    n5063 = local read "bin"() -> (w1874:dbl)
                    n5064 = local read "Override AI buffer"() -> (w1857:bool)
                    n5065 = local read "finite samples"() -> (w1883:bool)
                    n5066 = local read "srateAODOtt"() -> (w1870:dbl)
                    n5067 = local read "srateAODOtt"() -> (w1877:dbl)
                    n5068 = local read "continuous"() -> (w1882:bool)
                    n5069 = local read "Angle ref"() -> (w1867:dbl)
                    n5070 = local read "wavdet"() -> (w1884:bool)
                    n5071 = local read "Vx-ref"() -> (w1879:dbl)
                    n5072 = local read "Vy-ref"() -> (w1881:dbl)
                    n5073 = local read "avpp"() -> (w1880:i32)
                    n5074 = call "tt_timeandsamples.vi"("bin"=w1874, "refreshtime"=w1868, "srateAODOtt"=w1871, "tot#ofsamples"=w1876) -> ("refreshrate"=w1872:dbl, "refreshbuffer"=w1873:i32, "timetracecycles"=w1878:i32)  [unwired: 5 in]
                    n5075 = local read "bin"() -> (w1875:dbl)
                    n5076 = call "2pparameters.vi"("command"="get") -> ("params out"=w1887:T12)  [unwired: 1 in]
                    n5077 = Bundle By Name(cluster=w1887, "Drawing Mode"=w1860, "measpoints"=w1876, "tt_cycles"=w1878, "refreshbuffer"=w1873, "refreshrate"=w1872, "Vx-ref"=w1879, "Vy-ref"=w1881, "srate"=w1870, "finite"=w1883, "cont"=w1882, "wavdet"=w1884, "avpp"=w1880, "srateAODO"=w1877, "bufferAI"=w1873, "bin"=w1875, "Angle Img"=w1867, "Vxminref"=w1866, "Vxmaxref"=w1865, "Vyminref"=w1864, "Vymaxref"=w1863, "Xpixels Img"=w1862, "Ypixels Img"=w1861, "Pel"=w1859, "Vz-reset"=0.0, "AIoverride"=w1857, "type"="Lifetime (contour)") -> (w1885:T12)
                    n5078 = Reciprocal(x=w1872) -> (1/x=w1869:dbl)
                    n5079 = local write "refreshtime"(w1869) -> ()
                    n5080 = call "2pparameters.vi"("Params in"=w1885, "command"="set") -> ()  [unwired: 1 out]
                  }
                  frame "X-Y-Z-t movie" {
                  }
                  frame "linescan" {
                  }
                  frame "Timetrace" {
                    n5081 = local read "Vy-min draw"() -> (w1897:dbl)
                    n5082 = local read "Vy-max draw"() -> (w1896:dbl)
                    n5083 = local read "Vx-min draw"() -> (w1899:dbl)
                    n5084 = local read "Vx-max draw"() -> (w1898:dbl)
                    n5085 = local read "xpixels ref"() -> (w1895:i32)
                    n5086 = local read "ypixels ref"() -> (w1894:i32)
                    n5087 = local read "ROI Type"() -> (w1893:u16)
                    n5088 = local read "srateAODOtt"() -> (w1904:dbl)
                    n5089 = local read "# of frames"() -> (w1909:i32)
                    n5090 = local read "refreshtime"() -> (w1901:dbl)
                    n5091 = local read "Pel"() -> (w1892:dbl)
                    n5092 = local read "bin"() -> (w1907:dbl)
                    n5093 = local read "Override AI buffer"() -> (w1890:bool)
                    n5094 = local read "finite samples"() -> (w1916:bool)
                    n5095 = local read "srateAODOtt"() -> (w1903:dbl)
                    n5096 = local read "srateAODOtt"() -> (w1910:dbl)
                    n5097 = local read "continuous"() -> (w1915:bool)
                    n5098 = local read "Angle ref"() -> (w1900:dbl)
                    n5099 = local read "wavdet"() -> (w1917:bool)
                    n5100 = local read "Vx-ref"() -> (w1912:dbl)
                    n5101 = local read "Vy-ref"() -> (w1914:dbl)
                    n5102 = local read "avpp"() -> (w1913:i32)
                    n5103 = call "tt_timeandsamples.vi"("bin"=w1907, "refreshtime"=w1901, "srateAODOtt"=w1904, "tot#ofsamples"=w1909) -> ("refreshrate"=w1905:dbl, "refreshbuffer"=w1906:i32, "timetracecycles"=w1911:i32)  [unwired: 5 in]
                    n5104 = local read "bin"() -> (w1908:dbl)
                    n5105 = call "2pparameters.vi"("command"="get") -> ("params out"=w1920:T12)  [unwired: 1 in]
                    n5106 = Bundle By Name(cluster=w1920, "Drawing Mode"=w1893, "measpoints"=w1909, "tt_cycles"=w1911, "refreshbuffer"=w1906, "refreshrate"=w1905, "Vx-ref"=w1912, "Vy-ref"=w1914, "srate"=w1903, "finite"=w1916, "cont"=w1915, "wavdet"=w1917, "avpp"=w1913, "srateAODO"=w1910, "bufferAI"=w1906, "bin"=w1908, "Angle Img"=w1900, "Vxminref"=w1899, "Vxmaxref"=w1898, "Vyminref"=w1897, "Vymaxref"=w1896, "Xpixels Img"=w1895, "Ypixels Img"=w1894, "Pel"=w1892, "Vz-reset"=0.0, "AIoverride"=w1890, "type"="Timetrace") -> (w1918:T12)
                    n5107 = Reciprocal(x=w1905) -> (1/x=w1902:dbl)
                    n5108 = local write "refreshtime"(w1902) -> ()
                    n5109 = call "2pparameters.vi"("Params in"=w1918, "command"="set") -> ()  [unwired: 1 out]
                  }
                  frame "Lifetime (point)" {
                  }
                }
              }
              frame #1 {
                w1923 = FALSE ("wavdet")
                n5110 = call "2pparameters.vi"("command"="get") -> ("params out"=w1927:T12)  [unwired: 1 in]
                n5111 = Bundle By Name(cluster=w1927, "finite"=w1923, "cont"=w1923, "wavdet"=TRUE) -> (w1924:T12)
                n5112 = call "2pparameters.vi"("Params in"=w1924, "command"="set") -> ()  [unwired: 1 out]
              }
              frame #2 {
                n5113 = property on="Loaded settings" class="Ring (strict)"() -> ("RingText.Text"=w1929:string)  [unwired: 2 in, 2 out]
                n5114 = control-ref of="Analog Lines Plot"() -> (w1931:refnum<vi>)
                n5115 = control-ref of="Digital Lines Plot"() -> (w1930:refnum<vi>)
                n5116 = call "Usedlinesfromsettingsfile.vi"("sertting"=w1929) -> ("used AO names"=w1935:string[], "used AO lines"=w1934:tag[], "used DO names"=w1933:string[], "used DO lines"=w1932:tag[])
                n5117 = call "loadAODOwfparamsfromsettingsfile.vi"("sertting"=w1929) -> ()
                n5118 = call "prepAOWaveplot.vi"("WaveformGraph in"=w1931, "Analog Used Names"=w1935) -> ()  [unwired: 1 in]
                n5119 = local write "Analog Used Names"(w1935) -> ()
                n5120 = local write "Analog Used Lines"(w1934) -> ()
                n5121 = call "prepDOWaveplot.vi"("DigitalGraph in"=w1930, "used DO names"=w1933) -> ()  [unwired: 1 in]
                n5122 = local write "Digital Used Names"(w1933) -> ()
                n5123 = local write "Digital Used Lines"(w1932) -> ()
              }
              frame #3 {
                n5124 = call "waveformparamsv2.vi"("command"="get") -> ("Params out"=w1952:T16)  [unwired: 4 in, 2 out]
                n5125 = Unbundle By Name(w1952) -> ("AO parameters"=w1953:T17, "DO parameters"=w1954:T19)
                n5126 = for {
                  tunnel: w1953 -> [w1973] mode=indexing
                  tunnel: [w1971] -> w1955 mode=indexing
                  tunnel: [w1970] -> w1940 mode=indexing
                  tunnel: [w1968] -> w1943 mode=indexing
                  i -> [w1972]
                  n5127 = Unbundle By Name(w1973) -> ("AOtab"=w1974:dbl)
                  n5128 = case shown="0, Default" w1974 {
                    tunnel: w1973 -> [_ w1985 w1987 w1989]
                    tunnel: [_ w1984 w1986 w1988] -> w1969
                    frame -1 {
                    }
                    frame 0, Default {
                      n5129 = call "generateRampedSquareWave_fromAOparameters.vi"("AO params"=w1985) -> ("Waveform"=w1984:waveform(dbl))  [unwired: 1 out]
                    }
                    frame 1 {
                      n5130 = call "generateTriWave_fromAOparameters.vi"("AO params"=w1987) -> ("Waveform"=w1986:waveform(dbl))  [unwired: 1 out]
                    }
                    frame 2 {
                      n5131 = call "matlabAOwffromparam.vi"("Cluster"=w1989) -> ("Waveform"=w1988:waveform(dbl))  [unwired: 1 out]
                    }
                  }
                  n5132 = case shown="0" w1972 {
                    tunnel: [w1979 -1] -> w1971
                    tunnel: [w1978 w1982] -> w1970
                    tunnel: w1969 -> [w1978 w1982]
                    tunnel: [w1975 -1.0] -> w1968
                    frame 0 {
                      n5133 = Unbundle By Name(w1978) -> ("dt"=w1977:dbl, "Y"=w1980:dbl[])
                      n5134 = Reciprocal(x=w1977) -> (1/x=w1976:dbl)
                      n5135 = Array Size(array=w1980) -> (size(s)=w1979:i32)
                      n5136 = Round To Nearest(number=w1976) -> (nearest integer value=w1975:dbl)
                    }
                    frame 1, Default {
                    }
                  }
                }
                n5137 = Index Array(array=w1955, index=0) -> (element=w1957:i32)
                n5138 = Index Array(array=w1943, index=0) -> (element=w1942:dbl)
                n5139 = for {
                  tunnel: w1954 -> [w1962] mode=indexing
                  tunnel: [w1960] -> w1941 mode=indexing
                  tunnel: w1957 -> [w1959]
                  n5140 = Unbundle By Name(w1962) -> ("DOtab"=w1961:dbl)
                  n5141 = case shown="0, Default" w1961 {
                    tunnel: w1962 -> [w1965 w1967]
                    tunnel: w1959 -> [w1964 _]
                    tunnel: [w1963 w1966] -> w1960
                    frame 0, Default {
                      n5142 = call "simple digital from wf params.vi"("waveform params"=w1965, "number of samples"=w1964) -> ("digital waveform"=w1963:digitalwaveform)
                    }
                    frame 1 {
                      n5143 = call "matlabDOwffromparam.vi"("waveform params"=w1967) -> ("digital waveform"=w1966:digitalwaveform)
                    }
                  }
                }
                n5144 = property on="refwf" class="Ring (strict)"() -> ("RingText.Text"=w1945:string)  [unwired: 2 in, 2 out]
                n5145 = call "correctwaveformsizetemp.vi"("new sampling frequency (Hz)"=w1942, "start"=FALSE, "reference waveforms to"=w1945, "Analog waveforms in"=w1940, "stop"=FALSE, "Digital waveforms in"=w1941) -> ("analog wf out"=w1939:waveform(dbl)[], "Digital wf out"=w1938:digitalwaveform[], "measpoints"=w1936:i32)
                n5146 = local read "wavdet"() -> (w1937:bool)
                n5147 = case shown="True" w1937 {
                  tunnel: w1936 -> [_ w1958]
                  frame False {
                  }
                  frame True {
                    n5148 = local write "# of frames"(w1958) -> ()
                  }
                }
                n5149 = local write "Analog Lines Plot"(w1939) -> ()
                n5150 = local write "Digital Lines Plot"(w1938) -> ()
                n5151 = call "GetNumCamFramesv2.vi"("Digital Waveform Graph"=w1938) -> ("Numeric"=w1950:i32)  [unwired: 10 in]
                n5152 = call "waveformsAObuffer.vi"("AO wf in"=w1939, "command"="set") -> ()  [unwired: 1 out]
                n5153 = call "waveformsDObuffer.vi"("DO wf in"=w1938, "command"="set") -> ()  [unwired: 1 out]
                n5154 = local write "Total Camera Frames"(w1950) -> ()
              }
              frame #4 {
                n5155 = local read "AO channels"() -> (w1990:u32)
                n5156 = call "2pparameters.vi"("command"="get") -> ("params out"=w1992:T12)  [unwired: 1 in]
                n5157 = Unbundle By Name(w1992) -> ("aAO"=w1991:u32[])
                n5158 = Search 1D Array(1D array=w1991, element=w1990) -> (index of element=w1994:i32)  [unwired: 1 in]
                n5159 = Equal?(x=w1994, y=-1.0) -> (x = y?=w1995:bool)
                n5160 = case shown="False" w1995 {
                  tunnel: w1994 -> [w2020 _]
                  frame False {
                    n5161 = call "waveformparamsv2.vi"("command"="get") -> ("Params out"=w2003:T16)  [unwired: 4 in, 2 out]
                    n5162 = Unbundle By Name(w2003) -> ("AO parameters"=w2002:T17)
                    n5163 = Index Array(array=w2002, index=w2020) -> (element=w2019:T18)
                    n5164 = Unbundle By Name(w2019) -> ("AOtab"=w2000:dbl, "Repeats"=w2018:dbl, "Cycles"=w2017:dbl, "Start amplitude (V)"=w2016:dbl, "Baseline (V)"=w2015:dbl, "Step size (V)"=w2014:dbl, "DC (%)"=w2013:dbl, "Sampling frequency (Hz)"=w2012:dbl, "Period (ms)"=w2011:dbl, "Offset (V)"=w2010:dbl, "Amplitude (V)"=w2009:dbl, "Frequency"=w2008:dbl, "Tri Repeats"=w2007:dbl, "phase shift (ms)"=w2006:dbl, "Pulses"=w2005:dbl, "Tri phase"=w2001:dbl, "padding value"=w1997:dbl, "Matlab wave file"=w1998:path)
                    n5165 = To Unsigned Long Integer(number=w2000) -> (unsigned 32bit integer=w1999:u32)
                    n5166 = local write "Build analog waveform tabs"(w1999) -> ()
                    n5167 = local write "Matlab waveform path"(w1998) -> ()
                    n5168 = local write "phase shift (ms)"(w2006) -> ()
                    n5169 = local write "Repeats"(w2018) -> ()
                    n5170 = local write "Cycles"(w2017) -> ()
                    n5171 = local write "Amplitude (V)"(w2009) -> ()
                    n5172 = local write "Matlab padding value"(w1997) -> ()
                    n5173 = local write "Tri padding value"(w1997) -> ()
                    n5174 = local write "Start amplitude (V)"(w2016) -> ()
                    n5175 = local write "Tri Phase (s)"(w2001) -> ()
                    n5176 = local write "Period (ms)"(w2011) -> ()
                    n5177 = local write "Tri Repeats"(w2007) -> ()
                    n5178 = local write "Offset (V)"(w2010) -> ()
                    n5179 = local write "Frequency"(w2008) -> ()
                    n5180 = local write "Pulses"(w2005) -> ()
                    n5181 = local write "padding value"(w1997) -> ()
                    n5182 = local write "Sampling rate \ncurrent wf"(w2012) -> ()
                    n5183 = local write "Baseline (V)"(w2015) -> ()
                    n5184 = local write "Step size (V)"(w2014) -> ()
                    n5185 = local write "DC (%)"(w2013) -> ()
                  }
                  frame True {
                  }
                }
              }
              frame #5 {
                n5186 = local read "DO channels"() -> (w2023:u16)
                n5187 = call "2pparameters.vi"("command"="get") -> ("params out"=w2025:T12)  [unwired: 1 in]
                n5188 = Unbundle By Name(w2025) -> ("aDO"=w2024:u32[])
                n5189 = Search 1D Array(1D array=w2024, element=w2023) -> (index of element=w2022:i32)  [unwired: 1 in]
                n5190 = Equal?(x=w2022, y=-1.0) -> (x = y?=w2021:bool)
                n5191 = case shown="False" w2021 {
                  tunnel: w2022 -> [w2040 _]
                  frame False {
                    n5192 = call "waveformparamsv2.vi"("command"="get") -> ("Params out"=w2034:T16)  [unwired: 4 in, 2 out]
                    n5193 = Unbundle By Name(w2034) -> ("DO parameters"=w2032:T19)
                    n5194 = Index Array(array=w2032, index=w2040) -> (element=w2039:T20)
                    n5195 = Unbundle By Name(w2039) -> ("Digital DC (%)"=w2038:dbl, "Digital phase"=w2037:dbl, "Digital Freq (Hz)"=w2036:dbl, "Sampling frequency (Hz)"=w2035:dbl, "Digital time offset (s)"=w2031:dbl, "padding value"=w2030:dbl, "matlab wave file"=w2029:path, "DOtab"=w2028:dbl)
